vi "Generate Error.vi"(0 "code":i32, 1 "<append> (\"\")":string, 2 "<err> (\"\")":string, 5 "chain levels to remove (1)":i32=1 min=1, 9 "status (F)":bool, 11 "error in":errorcluster) -> (15 "error out":errorcluster)   [LabVIEW 2014, in "AMC.lvlib"]
uses:
  AMC.lvlib
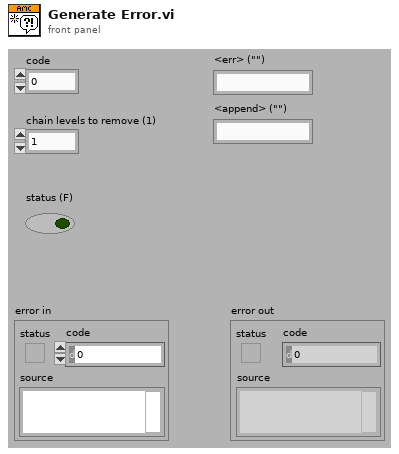
[diagram p1: front panel]
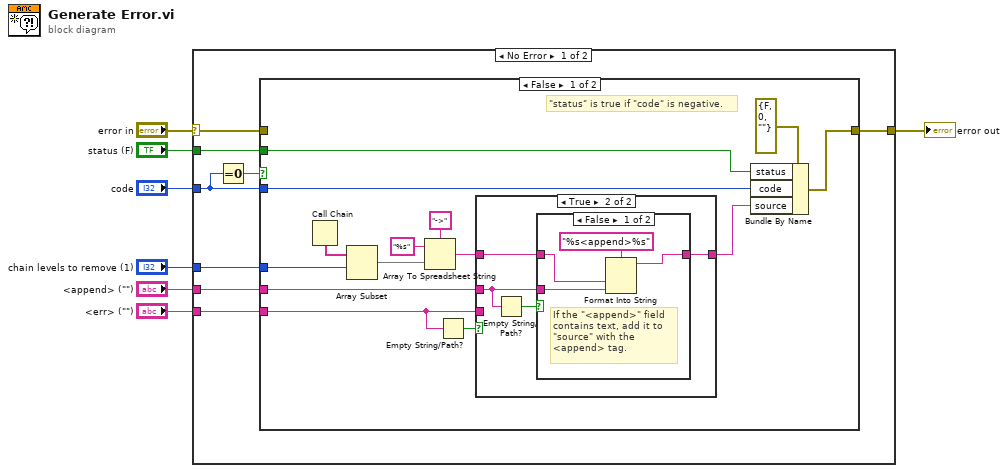
[diagram p0: block diagram]
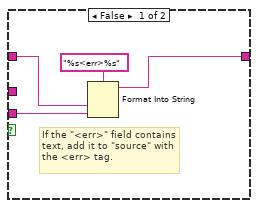
[diagram p2: hidden frame]
diagram:
  n1 = case shown="No Error" "error in" {
    selector: "error in" -> [w13 w44]
    tunnel: [w14 w44] -> w2
    tunnel: "code" -> [w12 _]
    tunnel: "chain levels to remove (1)" -> [w15 _]
    tunnel: "<err> (\"\")" -> [w11 _]
    tunnel: "<append> (\"\")" -> [w10 _]
    tunnel: "status (F)" -> [w8 _]
    frame No Error {
      n2 = Equal To 0?(x=w12) -> (x = 0?=w9:bool)
      n3 = case shown="False" w9 {
        tunnel: w13 -> [_ w43]
        tunnel: w15 -> [w28 _]
        tunnel: [w27 w43] -> w14
        tunnel: w12 -> [w23 _]
        tunnel: w11 -> [w20 _]
        tunnel: w10 -> [w19 _]
        tunnel: w8 -> [w16 _]
        frame False {
          # "\"status\" is true if \"code\" is negative."
          n4 = Call Chain() -> (call chain=w29:string[])
          n5 = Array Subset(array=w29, index=w28) -> (w26:string[])  [unwired: 1 in]
          n6 = Array To Spreadsheet String(delimiter (Tab)="->", array=w26, 3:"%s" ("format string")) -> (spreadsheet string=w22:string)
          n7 = Empty String/Path?(string/path=w20) -> (empty?=w21:bool)
          n8 = case shown="True" w21 {
            tunnel: w22 -> [w30 w35]
            tunnel: w20 -> [w31 _]
            tunnel: w19 -> [_ w36]
            tunnel: [w32 w34] -> w18
            frame False {
              # "If the \"<err>\" field contains text, add it to \"source\" with the <err> tag."
              n9 = Format Into String(format string="%s<err>%s", w30, w31) -> (resulting string=w32:string)  [unwired: 2 in, 1 out]
            }
            frame True {
              n10 = Empty String/Path?(string/path=w36) -> (empty?=w37:bool)
              n11 = case shown="False" w37 {
                tunnel: w36 -> [w40 _]
                tunnel: w35 -> [w41 w42]
                tunnel: [w38 w42] -> w34
                frame False {
                  # "If the \"<append>\" field contains text, add it to \"source\" with the <append> tag."
                  n12 = Format Into String(format string="%s<append>%s", w41, w40) -> (resulting string=w38:string)  [unwired: 2 in, 1 out]
                }
                frame True {
                }
              }
            }
          }
          n13 = Bundle By Name(cluster=errorcluster {"status"=FALSE, "code"=0, "source"=""} ("error IO"), "status"=w16, "code"=w23, "source"=w18) -> (w27:errorcluster)
        }
        frame True {
          # "Do nothing if the new code is zero."
        }
      }
    }
    frame Error {
      # "Do nothing if there is already an error on the wire."
    }
  }
  "error out" <- w2
